vi "STOP ECU Reading Process.vi"(8 "error in":errorcluster) -> (0 "error out":errorcluster, 3 "End of Communication":bool)   [LabVIEW 2024, in "RT Management.lvlib"]
uses:
  RT Management.lvlib
  ECU Internal Communications/Notifiers - Get.vi
  ECU Internal Communications/ECU InterComm.lvlib
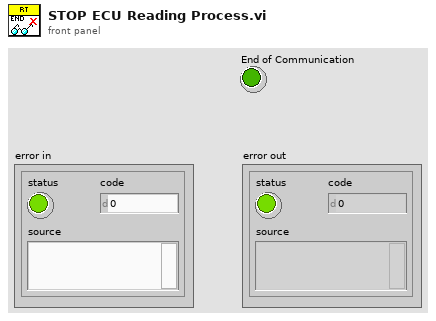
[diagram p1: front panel]
types:
  T1 = typedef "ECU InterComm.lvlib/ECU Notifiers.ctl" = cluster{"Tester Detected":refnum<notifier>, "STOP Reading":refnum<notifier>}
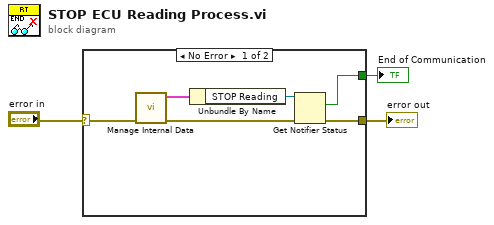
[diagram p0: block diagram]
diagram:
  n1 = case shown="No Error" "error in" {
    selector: "error in" -> [w6 w10]
    tunnel: [w4 w10] -> w3
    tunnel: [w5 _] -> w1
    frame No Error {
      n2 = call-poly "Manage Internal Data.vi"("error in"=w6) -> ("error out"=w9:errorcluster, "ECU Notifiers"=w7:T1)  [unwired: 9 in]
      n3 = Unbundle By Name(w7) -> ("STOP Reading"=w8:refnum<notifier>)
      n4 = Get Notifier Status(notifier=w8, error in (no error)=w9) -> (current notification=w5:bool, error out=w4:errorcluster)  [unwired: 3 out]
    }
    frame Error {
    }
  }
  "error out" <- w3
  "End of Communication" <- w1
